vi "PH_SHS_Analysis_Calibrator.PC Select Cam.vi"(0 "VI in":refnum<vi>, 2 "Source":string, 5 "error in (no error)":errorcluster) -> (14 "VI out":refnum<vi>, 19 "error out":errorcluster)   [LabVIEW 2014, in "PH_SHS_Analysis_Calibrator.lvlib"]
uses:
  PH_SHS_Analysis_Calibrator.lvlib
  CS_Core/BaseSM/BaseSM.lvlib
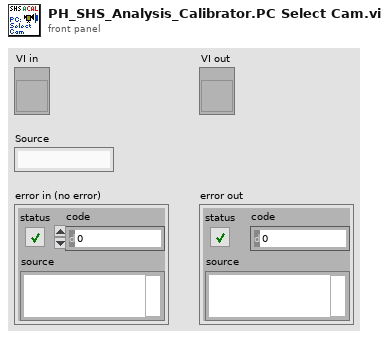
[diagram p1: front panel]
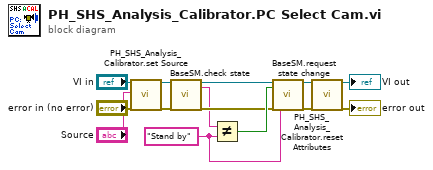
[diagram p0: block diagram]
diagram:
  w13 = "Stand by" ("y")
  n1 = call "PH_SHS_Analysis_Calibrator.set Source.vi"("i ref in"="VI in", "Source"="Source", "error in (no error)"="error in (no error)") -> ("i ref out"=w9:refnum<vi>, "error out"=w11:errorcluster)  [unwired: 15 in]
  n2 = call "BaseSM.check state.vi"("i ref in"=w9, "error in (no error)"=w11) -> ("i ref out"=w8:refnum<vi>, "actualState"=w6:string, "error out"=w7:errorcluster)  [unwired: 12 in, 3 out]
  n3 = Not Equal?(x=w6, y=w13) -> (x != y?=w14:bool)
  n4 = call "BaseSM.request state change.vi"("i ref in"=w8, "change"=w14, "error in (no error)"=w7, "requested state"=w13) -> ("i ref out"=w10:refnum<vi>, "error out"=w12:errorcluster)  [unwired: 12 in, 2 out]
  n5 = call "PH_SHS_Analysis_Calibrator.reset Attributes.vi"("i ref in"=w10, "error in (no error)"=w12) -> ("i ref out"=→"VI out":refnum<vi>, "error out"=→"error out":errorcluster)  [unwired: 16 in]
